vi "Write Data.vi"(8 "error in (no error)":errorcluster, 9 "Publication Time":timestamp, 10 "Value":variant, 11 "RingStringsBinding In":refnum<class "RingStringsBinding.lvclass">) -> (0 "error out":errorcluster, 3 "RingStringsBinding Out":refnum<class "RingStringsBinding.lvclass">)   [LabVIEW 2019, in "RingStringsBinding.lvclass"]
doc: "<License>\nCopyright © 2017 Composed Systems, LLC | All rights reserved\nwww.composed.io\n\nAuthor: Ethan Stern <ethan.stern@composed.io>\n\nThis software is provided \"AS IS\" WITHOUT WARRANTIES, either express or implied, AND IS FOR EDUCATIONAL PURPOSES ONLY.\n</License>MVA Framework 1.0.4.16\nEthan Stern - Composed Systems\nCopyright (c) 2017, Composed Systems"
uses:
  <vilib>/gpm_packages/@cs/transport/Source/Concrete/RingStringsBinding/RingStringsBinding.lvclass
  <vilib>/gpm_packages/@cs/transport/Source/Concrete/RingStringsBinding/RingStringsBinding.lvclass/RingStringsBinding.ctl
  <vilib>/Utility/error.llb/Error Cluster From Error Code.vi
  <vilib>/ErrorRing/Error Ring.xnode
  <vilib>/Utility/Data Type/NI_Data Type.lvlib
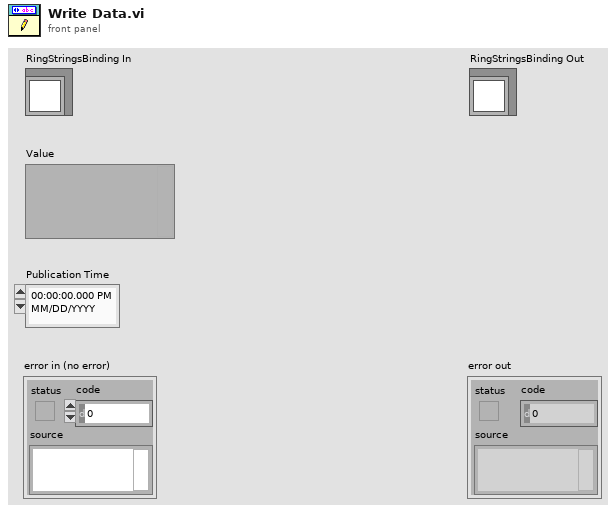
[diagram p1: front panel]
types:
  T1 = typedef "NI_Data Type.lvlib/Data Type.ctl" = enum8{"Invalid Type", "Void", "I8", "I16", "I32", "I64", "U8", "U16", "U32", "U64", "Single Float", "Double Float", "Extended Float", "Single Complex", "Double Complex", "Extended Complex", "Enum U8", "Enum U16", "Enum U32", "Enum U64", "Single Float With Unit", "Double Float With Unit", "Extended Float With Unit", "Single Complex with Unit", "Double Complex with Unit", "Extended Complex with Unit", "Boolean", "String", "Path", "Picture", "Tag", "Array", "Cluster", "Variant", "LV Variant", "Waveform", "Timestamp", "Digital Waveform", "Digital Data", "ExpressData", "Refnum", "External Data", "VI", "Poly VI", "LabVIEW Class Instance", "Fixed Point", "Set Collection", "Map Collection"}
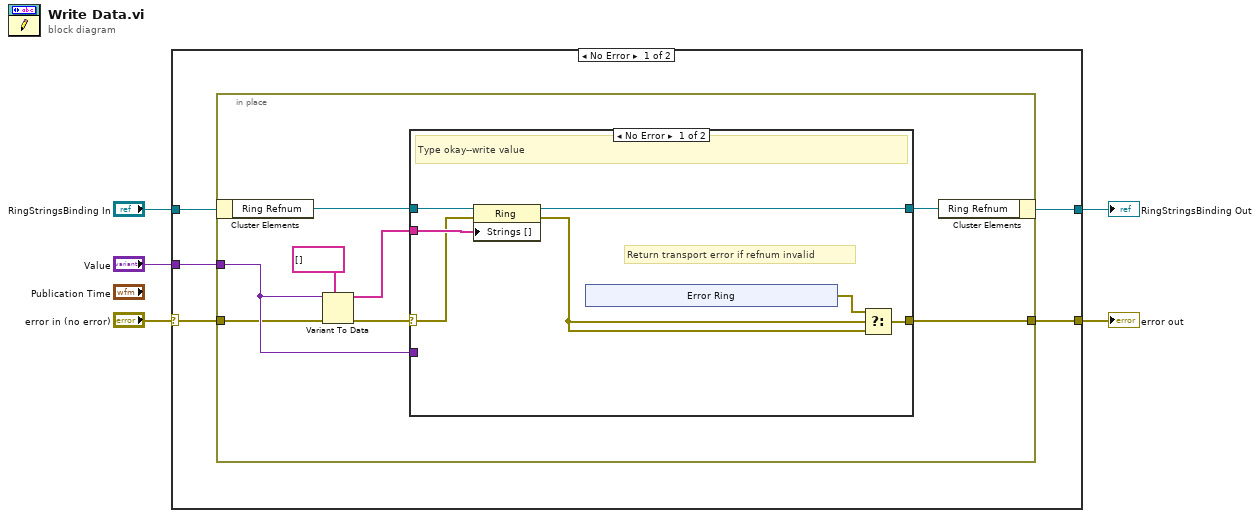
[diagram p0: block diagram]
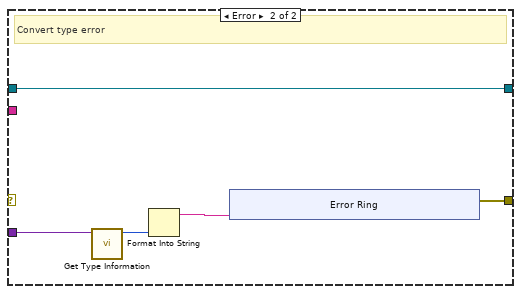
[diagram p2: hidden frame]
diagram:
  n1 = case shown="No Error" "error in (no error)" {
    selector: "error in (no error)" -> [w6 w44]
    tunnel: "Value" -> [w10 _]
    tunnel: [w9 w44] -> w4
    tunnel: "RingStringsBinding In" -> [w8 w43]
    tunnel: [w7 w43] -> w2
    frame No Error {
      n2 = in-place {
        in-place-border: w10 -> [w13]
        in-place-border: [w14] -> w9
        in-place-border: w6 -> [w11]
        n3 = in-place-cluster #1(w8) -> ("Ring Refnum"=w16:refnum<vi>)
        n4 = Variant To Data(error in=w11, type=string[] [] ("Strings []"), Variant=w13) -> (data=w17:string[], error out=w12:errorcluster)
        n5 = case shown="No Error" w12 {
          selector: w12 -> [w24 _]
          tunnel: w17 -> [w25 _]
          tunnel: w16 -> [w23 w35]
          tunnel: [w22 w35] -> w15
          tunnel: [w20 w33] -> w14
          tunnel: w13 -> [_ w34]
          frame No Error {
            # "Return transport error if refnum invalid"
            # "Type okay--write value"
            n6 = property class="Ring"(reference=w23, error in=w24, "Strings []"=w25) -> (reference out=w22:refnum<vi>, error out=w21:errorcluster)
            n7 = xnode "Error Ring"() -> ("error out"=w19:errorcluster)
            n8 = Select(t=w19, s=w21, f=w21) -> (s? t:f=w20:errorcluster)
          }
          frame Error {
            # "Convert type error"
            n9 = call <vilib>:"Get Type Information.vi"("variant"=w34) -> ("type"=w31:T1)  [unwired: 6 in, 4 out]
            n10 = Format Into String(w31) -> (resulting string=w32:string)  [unwired: 3 in, 1 out]
            n11 = xnode "Error Ring"("parameter 0"=w32) -> ("error out"=w33:errorcluster)
          }
        }
        n12 = in-place-cluster #1("Ring Refnum"=w15) -> (w7:refnum<class "RingStringsBinding.lvclass">)
      }
    }
    frame Error {
    }
  }
  "error out" <- w4
  "RingStringsBinding Out" <- w2
